vi "ActOnTrigOff.vi"(0 "ActionLvDialog in":refnum<class "ActionLvDialog.lvclass">, 1 "Data":variant, 5 "error in (no error)":errorcluster) -> (14 "ActionLvDialog out":refnum<class "ActionLvDialog.lvclass">, 19 "error out":errorcluster)   [LabVIEW 2017, in "ActionLvDialog.lvclass"]
doc: "Base class implementation (empty)."
uses:
  ActionLvDialog.lvclass
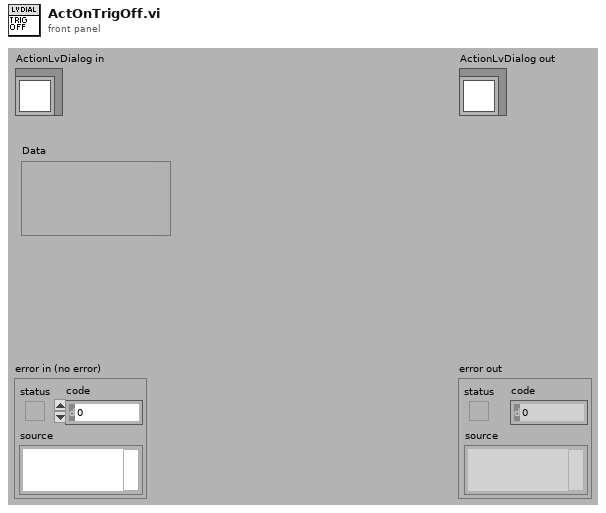
[diagram p1: front panel]
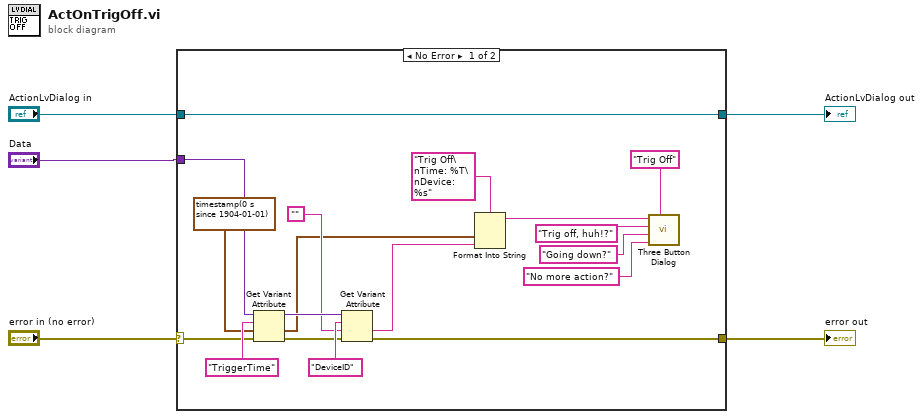
[diagram p0: block diagram]
diagram:
  n1 = case shown="No Error" "error in (no error)" {
    selector: "error in (no error)" -> [w16 w24]
    tunnel: "ActionLvDialog in" -> [w23 w25]
    tunnel: [w23 w25] -> w4
    tunnel: [w9 w24] -> w2
    tunnel: "Data" -> [w15 _]
    frame No Error {
      n2 = Get Variant Attribute(Variant=w15, name="TriggerTime", default value (empty Variant)=timestamp(0 s since 1904-01-01) ("TriggerTime"), error in=w16) -> (duplicate Variant=w18:variant, value=w12:timestamp, error out=w19:errorcluster)  [unwired: 1 out]
      n3 = Get Variant Attribute(Variant=w18, name="DeviceID", default value (empty Variant)="", error in=w19) -> (value=w11:string, error out=w9:errorcluster)  [unwired: 2 out]
      n4 = Format Into String(format string="Trig Off\nTime: %T\nDevice: %s", w12, w11) -> (resulting string=w10:string)  [unwired: 2 in, 1 out]
      n5 = call <vilib>:"Three Button Dialog.vi"("Window Title (\"\")"="Trig Off" ("Window Title (\"\")"), "Right Button Text (\"Cancel\")"="No more action?" ("Left Button Text (\"Yes\")"), "Center Button Text (\"No\")"="Going down?" ("Left Button Text (\"Yes\")"), "Left Button Text (\"Yes\")"="Trig off, huh!?" ("Left Button Text (\"Yes\")"), "message"=w10) -> ()  [unwired: 6 in, 1 out]
    }
    frame Error {
    }
  }
  "error out" <- w2
  "ActionLvDialog out" <- w4
